vi "Configure Trigger Model LAN Output Protocol.vi"(8 "error in (no error)":errorcluster, 9 "Protocol (TCP)":u16(ring) items=["TCP", "UDP", "Multicast"], 10 "LAN Event Number   (1)":i32=1 min=1 max=8 step=1 format="%#.6g", 11 "VISA resource name":refnum<visa-resource-name>) -> (0 "error out":errorcluster, 3 "VISA resource name out":refnum<visa-resource-name>)   [LabVIEW 2022 SP3, in "Keithley 2450.lvlib"]
doc: "This VI sets the LAN protocol to use for sending trigger messages."
uses:
  Keithley 2450.lvlib
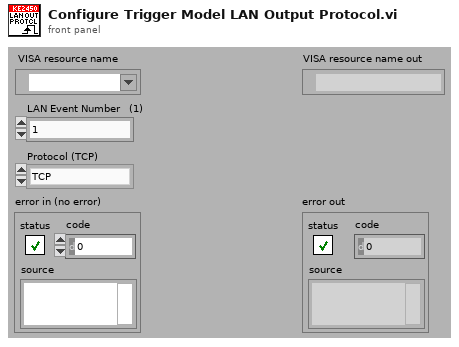
[diagram p1: front panel]
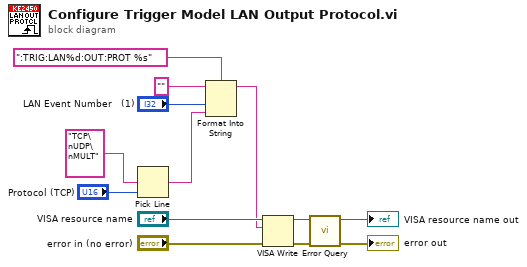
[diagram p0: block diagram]
diagram:
  n1 = Pick Line(multi-line string="TCP\nUDP\nMULT", line index="Protocol (TCP)") -> (output string=w1:string)  [unwired: 1 in]
  n2 = Format Into String(format string=":TRIG:LAN%d:OUT:PROT %s", initial string="", "LAN Event Number   (1)", w1) -> (resulting string=w4:string)  [unwired: 1 in, 1 out]
  n3 = VISA Write(VISA resource name="VISA resource name", write buffer=w4, error in (no error)="error in (no error)") -> (VISA resource name out=w9:refnum<visa-resource-name>, error out=w8:errorcluster)  [unwired: 1 out]
  n4 = call "Error Query.vi"("error in (no error)"=w8, "VISA resource name"=w9) -> ("error out"=→"error out":errorcluster, "VISA resource name out"=→"VISA resource name out":refnum<visa-resource-name>)  [unwired: 8 out]
